vi "SetUI.vi"(0 "reference in":refnum<class "GUI.lvclass">, 5 "UI VI":refnum<vi>, 11 "error in (no error)":errorcluster) -> (4 "reference out":refnum<class "GUI.lvclass">, 15 "error out":errorcluster)   [LabVIEW 2019, in "GUI.lvclass"]
uses:
  GUI.lvclass
  GUI.lvclass/GUI.ctl
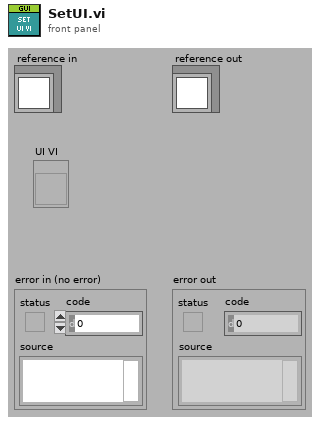
[diagram p1: front panel]
types:
  T1 = typedef "GUI.lvclass/Shered Data.ctl" = cluster{"WindowsState":T2, "UI VI":refnum<vi>, "SubPnl":refnum<vi>}
  T2 = typedef "GUI.lvclass/WindowsState.ctl" = enum16{"NotReady", "Ready", "Inserted", "Opened"}
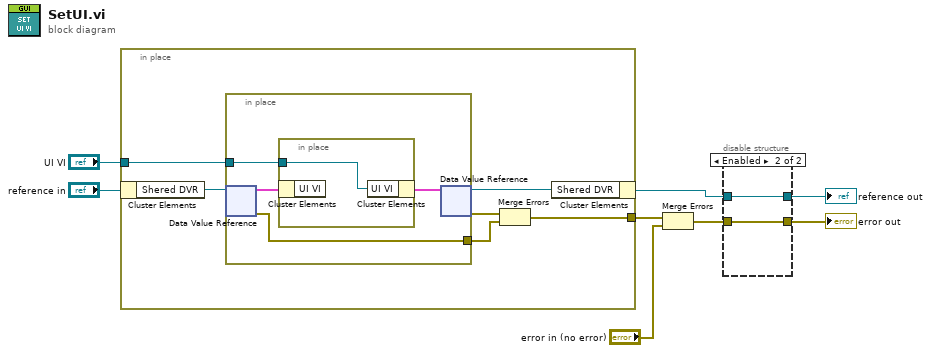
[diagram p0: block diagram]
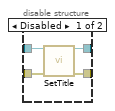
[diagram p2: hidden frame]
diagram:
  n1 = in-place {
    in-place-border: "UI VI" -> [w10]
    in-place-border: [w9] -> w1
    n2 = in-place-cluster #1("reference in") -> ("Shered DVR"=w14:refnum<data-value>)
    n3 = in-place {
      in-place-border: [w16] -> w11
      in-place-border: w10 -> [w15]
      n4 = in-place-dvr #2(w14) -> (w18:T1, w16:errorcluster)
      n5 = in-place {
        in-place-border: w15 -> [w19]
        n6 = in-place-cluster #3(w18) -> ()  [unwired: 1 out]
        n7 = in-place-cluster #3("UI VI"=w19) -> (w17:T1)
      }
      n8 = in-place-dvr #2(w17) -> (w13:refnum<data-value>, w12:errorcluster)
    }
    n9 = Merge Errors(w12, w11) -> (w9:errorcluster)
    n10 = in-place-cluster #1("Shered DVR"=w13) -> (w4:refnum<class "GUI.lvclass">)
  }
  n11 = Merge Errors(w1, "error in (no error)") -> (w2:errorcluster)
  n12 = disable-structure shown="Enabled" {
    disable-tunnel: [w23 w25] -> w7
    disable-tunnel: [w22 w24] -> w6
    disable-tunnel: w4 -> [w21 w25]
    disable-tunnel: w2 -> [w20 w24]
    frame Disabled {
      n13 = call "SetTitle.vi"("reference in"=w21, "error in (no error)"=w20) -> ("reference out"=w23:refnum<class "GUI.lvclass">, "error out"=w22:errorcluster)  [unwired: 12 in]
    }
    frame Enabled {
    }
  }
  "error out" <- w6
  "reference out" <- w7
